vi "setSerialNumber.vi"(8 "error in (no error)":errorcluster, 10 "serialNumber":string, 11 "CQT_DDS in":refnum<class "CQT_DDS.lvclass">) -> (0 "error out":errorcluster, 3 "CQT_DDS out":refnum<class "CQT_DDS.lvclass">)   [LabVIEW 2009, in "Hardware.lvlib" / "Channels.lvlib" / "CQT_DDS.lvclass"]
uses:
  CQT_DDS.lvclass
  CQT_DDS.lvclass/CQT_DDS.ctl
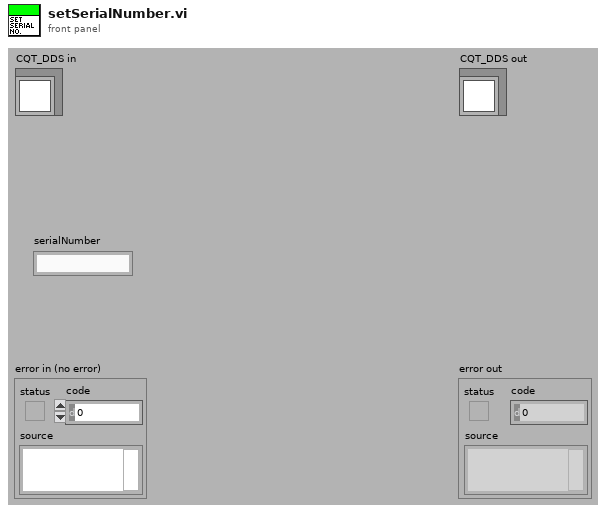
[diagram p1: front panel]
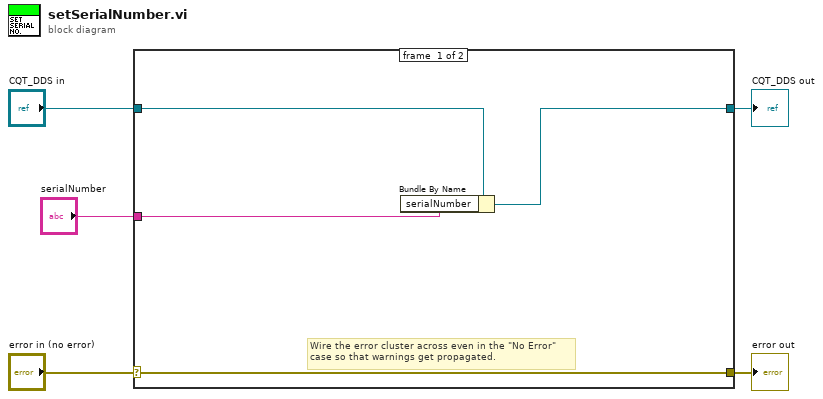
[diagram p0: block diagram]
diagram:
  n1 = case shown="No Error" "error in (no error)" {
    selector: "error in (no error)" -> [w9 w11]
    tunnel: [w9 w11] -> w4
    tunnel: [w7 w10] -> w2
    tunnel: "CQT_DDS in" -> [w8 w10]
    tunnel: "serialNumber" -> [w6 _]
    frame #0 {
      # "Wire the error cluster across even in the \"No Error\"\ncase so that warnings get propagated."
      n2 = Bundle By Name(cluster=w8, "serialNumber"=w6) -> (w7:refnum<class "CQT_DDS.lvclass">)
    }
    frame #1 {
    }
  }
  "error out" <- w4
  "CQT_DDS out" <- w2
